vi "DSF.Engine.Memory.ObjectPool.Get Objects.vi"(8 "error in (no error)":errorcluster, 11 "ObjectPool in":refnum<class "DSF.Engine.Memory.ObjectPool.lvclass">) -> (0 "error out":errorcluster, 2 "Objects":refnum<class>[](array[class]), 3 "ObjectPool out":refnum<class "DSF.Engine.Memory.ObjectPool.lvclass">)   [LabVIEW 2016, in "DSF.Engine.lvlib" / "DSF.Engine.Memory.ObjectPool.lvclass"]
uses:
  DSF.Engine.Memory.ObjectPool.lvclass
  DSF.Engine.Memory.ObjectPool.lvclass/DSF.Engine.Memory.ObjectPool.ctl
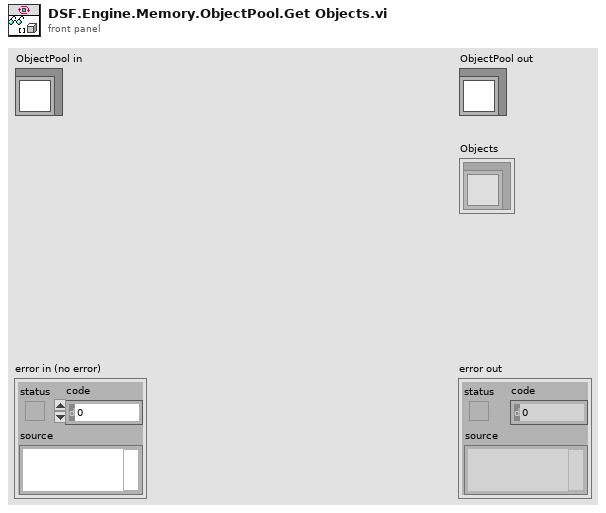
[diagram p1: front panel]
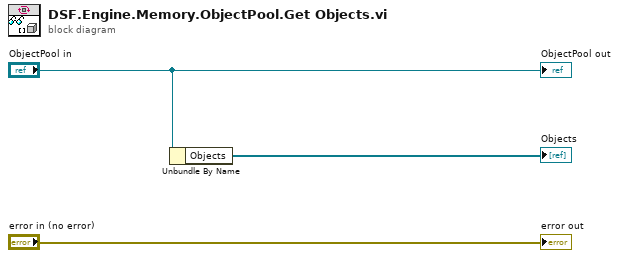
[diagram p0: block diagram]
diagram:
  n1 = Unbundle By Name("ObjectPool in") -> ("Objects"=→"Objects":refnum<class>[])
  "error out" <- "error in (no error)"
  "ObjectPool out" <- "ObjectPool in"
